vi "WriteFileDAQ.vi"(0 "DAQ File Name":string, 3 "error in":errorcluster) -> (7 "tdms file out":refnum<k34>, 10 "error out":errorcluster)   [LabVIEW 2020]
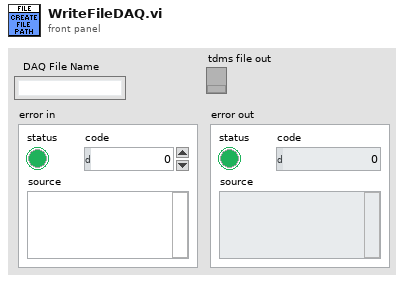
[diagram p1: front panel]
types:
  T1 = enum16{"open", "open or create", "create or replace", "create", "open (read-only)"}
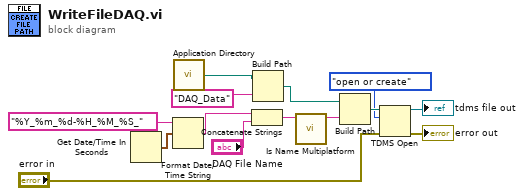
[diagram p0: block diagram]
diagram:
  n1 = Get Date/Time In Seconds() -> (seconds since 1Jan1904=w1:timestamp)
  n2 = Format Date/Time String(time format string (%c)="%Y_%m_%d-%H_%M_%S_", seconds (now)=w1) -> (date/time string=w13:string)  [unwired: 1 in]
  n3 = call <vilib>:"Application Directory.vi"() -> ("Application Directory"=w8:path)
  n4 = Concatenate Strings(w13, "DAQ File Name") -> (w4:string)
  n5 = Build Path(base path=w8, name or relative path="DAQ_Data") -> (appended path=w7:path)
  n6 = call <vilib>:"Is Name Multiplatform.vi"("filename"=w4) -> ("suggested filename"=w3:string)  [unwired: 6 in, 4 out]
  n7 = Build Path(base path=w7, name or relative path=w3) -> (appended path=w11:path)
  n8 = TDMS Open(8:"error in", 10:T1."open or create" ("operation (0:open)"), 11:w11) -> (0:→"error out":errorcluster, 3:→"tdms file out":refnum<k34>)  [unwired: 4 in]
